vi "CC Rd Wr Hardware Configuration.vi"(8 "error in (no error)":errorcluster, 10 "Write? (F:Read)":bool, 11 "Hardware Config":T1) -> (0 "error out":errorcluster, 2 "File":path, 3 "Hardware Config out":T1)   [LabVIEW 2021]
uses:
  typedefs/CC cluster Hardware Config.ctl
  typedefs/CC cluster Device Index.ctl
  2e80df6d-94aa-46b9-8b94-ceea8c057880.vi
  659fb017-0e9f-42f9-b06e-930303f00cbc.vi
  <vilib>/JDP Science/JSONtext/Find Item.vi
  <vilib>/JDP Science/JSONtext/Next JSON Value.vi
  <vilib>/JDP Science/JSONtext/String Subset.vi
  <vilib>/JDP Science/JSONtext/Parsing/Advance past next JSON Value (inlined COPY).vi
  <vilib>/JDP Science/JSONtext/Parsing/Advance past whitespace.vi
  <vilib>/JDP Science/JSONtext/Parsing/Advance past String.vi
  <vilib>/JDP Science/JSONtext/Parsing/Advance past Number.vi
  <vilib>/JDP Science/JSONtext/Parsing/Advance past Line Ending.vi
  <vilib>/JDP Science/JSONtext/Parsing/Parse Full Path or Item Name.vi
  <vilib>/JDP Science/JSONtext/Parsing/Advance past Array.vi
  <vilib>/JDP Science/JSONtext/Parsing/Advance past Object.vi
  <vilib>/JDP Science/JSONtext/support/Error Cluster From Code.vi
  <vilib>/JDP Science/JSONtext/Offset/Find Item Locations by Path.vi
  <vilib>/JDP Science/JSONtext/JSON text to Variant.vi
  <vilib>/JDP Science/JSONtext/Variant to JSON Text.vi
  <vilib>/JDP Science/JSONtext/Set Item.vi
  <vilib>/JDP Science/JSONtext/LVClass Serializer/JSONtext LVClass Serializer.lvclass
panel:
  in  "Settings File":string="CC System Settings.json"
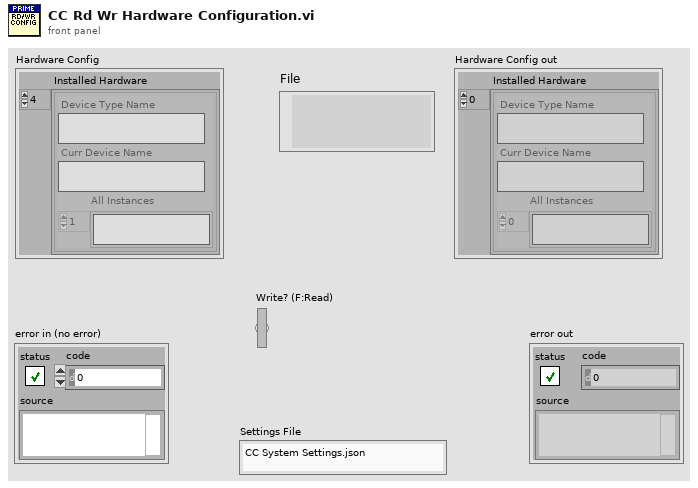
[diagram p1: front panel]
types:
  T1 = typedef "CC cluster Hardware Config.ctl" = cluster{"Installed Hardware":T2[]}
  T2 = typedef "CC cluster Device Index.ctl" = cluster{"Device Type Name":string, "Curr Device Name":string, "All Instances":string[]}
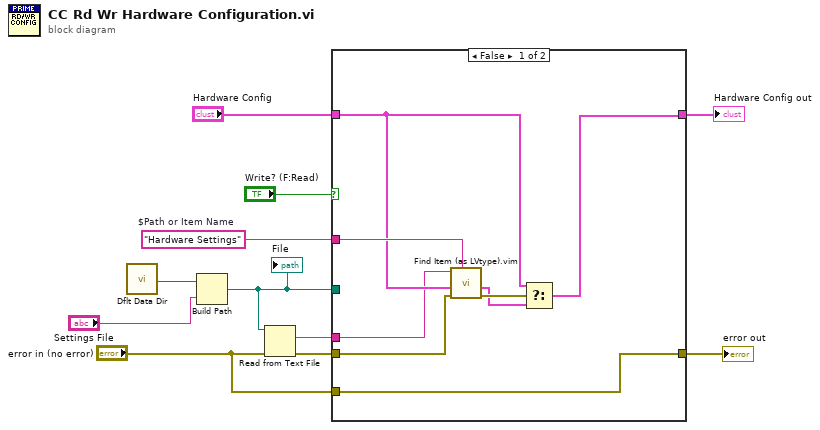
[diagram p0: block diagram]
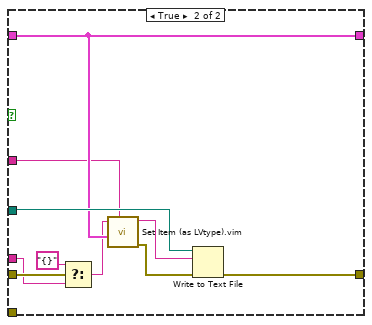
[diagram p2: hidden frame]
diagram:
  w5 = "Hardware Settings"  # $Path or Item Name
  n1 = call <vilib>:"Dflt Data Dir.vi"() -> ("App:Default Data Directory"=w9:path)
  n2 = Build Path(base path=w9, name or relative path="Settings File") -> (appended path=w2:path)
  "File" <- w2
  n3 = Read from Text File(file (use dialog)=w2, error in="error in (no error)") -> (text=w3:string, error out=w4:errorcluster)  [unwired: 2 in, 2 out]
  n4 = case shown="False" "Write? (F:Read)" {
    tunnel: w4 -> [w13 w24]
    tunnel: "Hardware Config" -> [w17 w27]
    tunnel: w2 -> [_ w29]
    tunnel: [w12 w28] -> w8
    tunnel: [w19 w27] -> w7
    tunnel: w5 -> [w18 w26]
    tunnel: w3 -> [w14 w22]
    tunnel: "error in (no error)" -> [w12 _]
    frame False {
      n5 = call "Find Item (as LVtype).vim"("$Path or Item Name"=w18, "error in (no error)"=w13, "Data Type and Default Value"=w17, "JSON"=w14) -> ("error out"=w16:errorcluster, "Data"=w15:T1)  [unwired: 4 in, 2 out]
      n6 = Select(t=w17, s=w16, f=w15) -> (s? t:f=w19:T1)
    }
    frame True {
      n7 = Select(t="{}" ("JSON"), s=w24, f=w22) -> (s? t:f=w21:string)
      n8 = call "Set Item (as LVtype).vim"("$Path or Item Name"=w26, "Anything"=w27, "JSON"=w21) -> ("error out"=w20:errorcluster, "<JSON>"=w25:string)  [unwired: 5 in, 1 out]
      n9 = Write to Text File(file (use dialog)=w29, text=w25, error in=w20) -> (error out=w28:errorcluster)  [unwired: 1 in, 2 out]
    }
  }
  "error out" <- w8
  "Hardware Config out" <- w7
